vi "Log Status Update.vi"(8 "error in (no error)":errorcluster, 10 "Status String":string, 11 "Cap Bank Server in":refnum<class "Cap Bank Server.lvclass">) -> (0 "error out":errorcluster, 3 "Cap Bank Server out":refnum<class "Cap Bank Server.lvclass">)   [LabVIEW 2015, in "Cap Bank Server.lvclass"]
uses:
  Cap Bank Server.lvclass
  Cap Bank Server.lvclass/Cap Bank Server.ctl
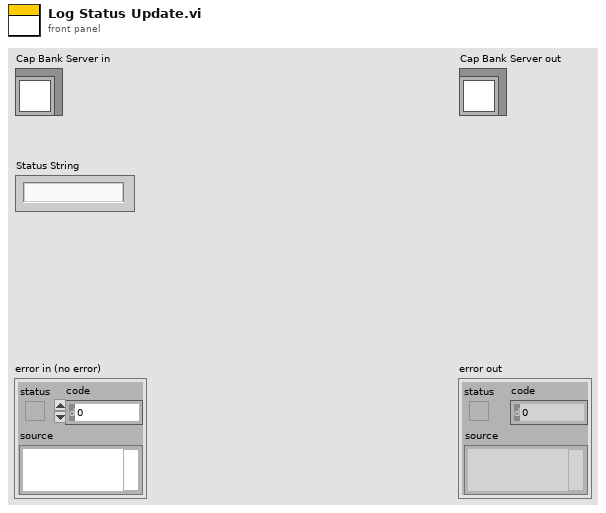
[diagram p1: front panel]
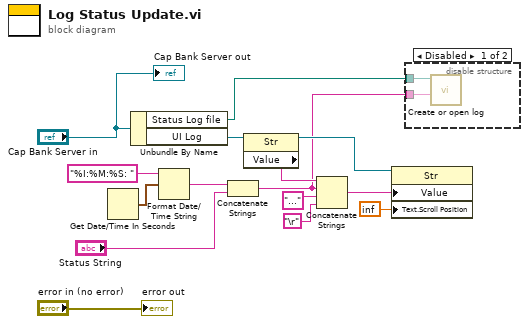
[diagram p0: block diagram]
diagram:
  n1 = Get Date/Time In Seconds() -> (seconds since 1Jan1904=w13:timestamp)
  n2 = Unbundle By Name("Cap Bank Server in") -> ("Status Log file"=w3:path, "UI Log"=w7:refnum<vi>)
  n3 = Format Date/Time String(time format string (%c)="%I:%M:%S: ", seconds (now)=w13) -> (date/time string=w15:string)  [unwired: 1 in]
  n4 = Concatenate Strings(w15, "Status String") -> (w1:string)
  n5 = property class="Str"(reference=w7) -> (reference out=w8:refnum<vi>, "Value"=w9:string)  [unwired: 1 in, 1 out]
  n6 = Concatenate Strings(w9, w1, "..." ("string"), "\r") -> (w2:string)
  n7 = property class="Str"(reference=w8, "Value"=w2, "Text.Scroll Position"=inf) -> ()  [unwired: 1 in, 2 out]
  n8 = disable-structure shown="Disabled" {
    disable-tunnel: w3 -> [w17 _]
    disable-tunnel: w1 -> [w16 _]
    frame Disabled {
      n9 = call "Create or open log.vi"("Log string"=w16, "appended path"=w17) -> ()  [unwired: 8 in, 2 out]
    }
    frame Enabled {
    }
  }
  "error out" <- "error in (no error)"
  "Cap Bank Server out" <- "Cap Bank Server in"
